vi "Core Stop Core.vi"(8 "error in (no error)":errorcluster, 11 "Instrument Sequencer in":refnum<class "Instrument Sequencer.lvclass">) -> (0 "error out":errorcluster, 3 "Instrument Sequencer out":refnum<class "Instrument Sequencer.lvclass">)   [LabVIEW 2020, in "Instrument Handler.lvlib" / "Instrument Sequencer.lvclass"]
doc: "The default implementation of this VI does nothing.\nUse this VI to terminate everything started in 'Pre Launch Init'."
uses:
  Instrument Sequencer.lvclass
  Instrument Sequencer.lvclass/Instrument Sequencer.ctl
  PPL/HDH.Actor Framework.Core.Instrument Driver.lvlibp/Instrument Driver/Instrument Driver.lvclass
  PPL/HDH.Actor Framework.Core.Sequencer.lvlibp/Sequencer Core/Sequencer Core.lvclass
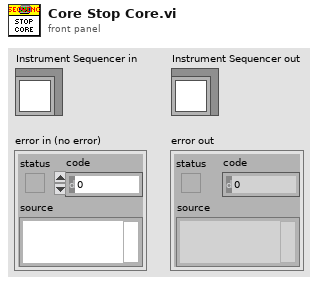
[diagram p1: front panel]
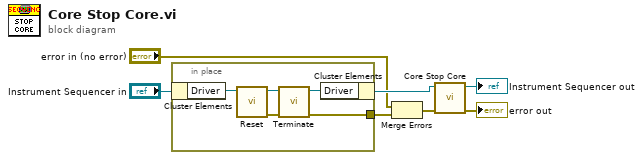
[diagram p0: block diagram]
diagram:
  n1 = in-place {
    in-place-border: [w8] -> w2
    n2 = in-place-cluster #1("Instrument Sequencer in") -> ("Driver"=w12:refnum<class "Instrument Driver.lvclass">)
    n3 = call "Reset.vi"("Instrument in"=w12) -> ("error out"=w9:errorcluster, "Instrument out"=w11:refnum<class "Instrument Driver.lvclass">)  [unwired: 9 in]
    n4 = call-dynamic "Terminate.vi"("error in (no error)"=w9, "Instrument in"=w11) -> ("error out"=w8:errorcluster, "Instrument out"=w10:refnum<class "Instrument Driver.lvclass">)  [unwired: 8 in]
    n5 = in-place-cluster #1("Driver"=w10) -> (w4:refnum<class "Instrument Sequencer.lvclass">)
  }
  n6 = Merge Errors("error in (no error)", w2) -> (w1:errorcluster)
  n7 = call-parent "Core Stop Core.vi"("error in (no error)"=w1, "Sequencer Core in"=w4) -> ("error out"=→"error out":errorcluster, "Sequencer Core out"=→"Instrument Sequencer out":refnum<class "Instrument Sequencer.lvclass">)  [unwired: 8 in]
